vi "MFC error alert sub vi.vi"() -> ()   [LabVIEW 2024]
uses:
  <vilib>/smtpClient/Set Message Text.vi
  <vilib>/smtpClient/LabVIEWSMTPClient.lvlib
panel:
  out "invalid recipients":string[](array[string])
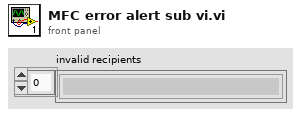
[diagram p1: front panel]
types:
  T1 = typedef "LabVIEWSMTPClient.lvlib/SmtpClientHandle.ctl" = refnum<k1>
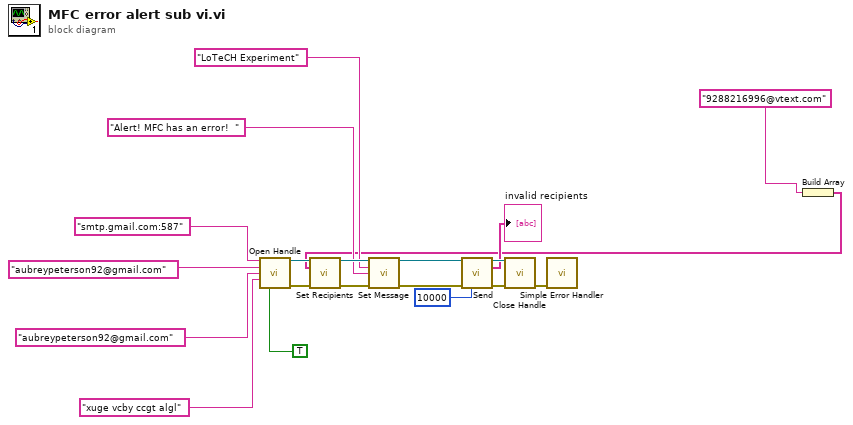
[diagram p0: block diagram]
diagram:
  n1 = call <vilib>:"Open Handle.vi"("server address"="smtp.gmail.com:587", "from"="aubreypeterson92@gmail.com", "username"="aubreypeterson92@gmail.com", "password"="xuge vcby ccgt algl", "use TLS (false)"=TRUE) -> ("handle out"=w16:T1, "error out"=w20:errorcluster)  [unwired: 9 in]
  n2 = Build Array("9288216996@vtext.com") -> (w1:string[])
  n3 = call <vilib>:"Set Recipients.vi"("handle in"=w16, "to"=w1, "error in (no error)"=w20) -> ("handle out"=w15:T1, "error out"=w19:errorcluster)  [unwired: 11 in]
  n4 = call-poly <vilib>:"Set Message.vi"("handle in"=w15, "subject"="LoTeCH Experiment", "plain text message"="Alert! MFC has an error!  ", "error in (no error)"=w19) -> ("handle out"=w14:T1, "error out"=w18:errorcluster)  [unwired: 10 in]
  n5 = call <vilib>:"Send.vi"("handle in"=w14, "error in (no error)"=w18, "timeout in ms (10000)"=10000) -> ("handle out"=w13:T1, "invalid recipients"=→"invalid recipients":string[], "error out"=w17:errorcluster)  [unwired: 10 in]
  n6 = call <vilib>:"Close Handle.vi"("handle in"=w13, "error in (no error)"=w17) -> ("error out"=w12:errorcluster)  [unwired: 12 in, 1 out]
  n7 = call <vilib>:"Simple Error Handler.vi"("error in (no error)"=w12) -> ()  [unwired: 4 in, 5 out]
